vi "Post Value.vi"(7 "PV name":string, 8 "error in":errorcluster, 10 "value pointer":i64, 11 "Server in":refnum<class "Server.lvclass">) -> (0 "error out":errorcluster, 3 "Server out":refnum<class "Server.lvclass">)   [LabVIEW 2020, in "Server.lvlib" / "Server.lvclass"]
uses:
  Server.lvclass
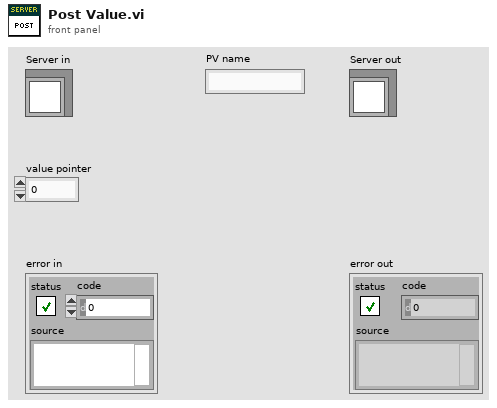
[diagram p1: front panel]
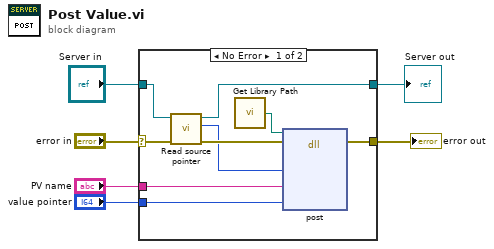
[diagram p0: block diagram]
diagram:
  n1 = case shown="No Error" "error in" {
    selector: "error in" -> [w15 w17]
    tunnel: [w12 w17] -> w4
    tunnel: [w9 w16] -> w5
    tunnel: "Server in" -> [w14 w16]
    tunnel: "PV name" -> [w8 _]
    tunnel: "value pointer" -> [w7 _]
    frame No Error {
      n2 = call "Read source pointer.vi"("error in (no error)"=w15, "Server in"=w14) -> ("error out"=w13:errorcluster, "source pointer"=w10:i64, "Server out"=w9:refnum<class "Server.lvclass">)  [unwired: 7 in]
      n3 = call "Get Library Path.vi"() -> ("Path"=w11:path)  [unwired: 1 in]
      n4 = dll-call lib="?" fn="post"(path in=w11, error in=w13, "source"=w10, "pv_name"=w8, "value"=w7) -> (error out=w12:errorcluster)  [unwired: 5 in, 1 out]
    }
    frame Error {
    }
  }
  "error out" <- w4
  "Server out" <- w5
